vi "Escape Brackets.vi"(1 "Pattern":string) -> (0 "result string":string)   [LabVIEW 2019, in "ProjectItem.lvclass"]
uses:
  ProjectItem.lvclass
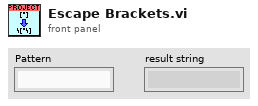
[diagram p1: front panel]
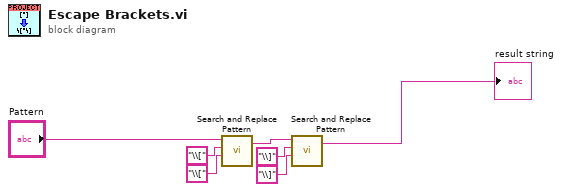
[diagram p0: block diagram]
diagram:
  n1 = call <vilib>:"Search and Replace Pattern.vi"("string"="Pattern", "regular expression (\"\")"="\\[" ("regular expression (\"\")"), "replace string (\"\")"="\\[" ("replace string (\"\")")) -> ("result string"=w5:string)  [unwired: 2 in, 1 out]
  n2 = call <vilib>:"Search and Replace Pattern.vi"("string"=w5, "regular expression (\"\")"="\\]" ("regular expression (\"\")"), "replace string (\"\")"="\\]" ("replace string (\"\")")) -> ("result string"=→"result string":string)  [unwired: 2 in, 1 out]
